vi "Generate Unique Random Name.vi"(8 "error in (no error)":errorcluster, 11 "Main in":refnum<class "Main.lvclass">) -> (0 "error out":errorcluster, 2 "Name":string, 3 "Main out":refnum<class "Main.lvclass">)   [LabVIEW 2020, in "Main.lvclass"]
uses:
  Main.lvclass
  Main.lvclass/Main.ctl
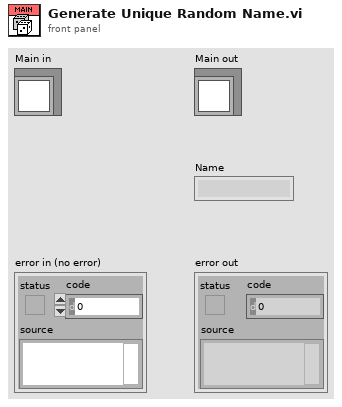
[diagram p1: front panel]
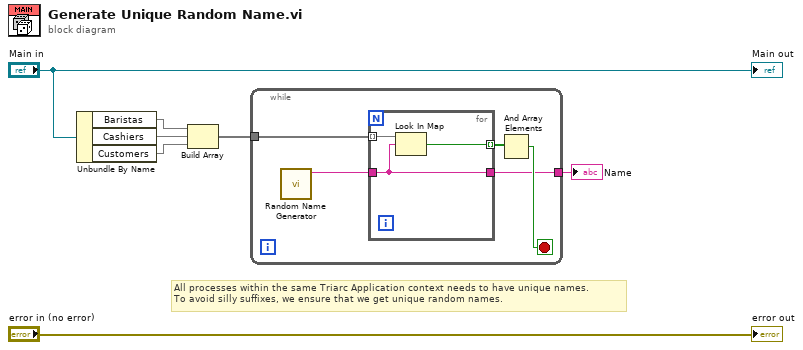
[diagram p0: block diagram]
diagram:
  # "All processes within the same Triarc Application context needs to have unique names.\nTo avoid silly suffixes, we ensure that we get unique random names."
  n1 = Unbundle By Name("Main in") -> ("Baristas"=w5:map{string, string}, "Cashiers"=w4:map{string, string}, "Customers"=w3:map{string, string})
  n2 = Build Array(w5, w4, w3) -> (w2:map{string, string}[])
  n3 = while {
    tunnel: w2 -> [w12]
    tunnel: [w8] -> w1
    stop <- w9 stop-if-true
    n4 = call "Random Name Generator.vi"() -> ("Name"=w11:string)  [unwired: 11 in]
    n5 = for {
      tunnel: w12 -> [w15] mode=indexing
      tunnel: w11 -> [w13]
      tunnel: [w14] -> w10 mode=indexing
      tunnel: [w13] -> w8
      n6 = Look In Map(map=w15, key=w13) -> (key not found?=w14:bool)  [unwired: 1 in, 1 out]
    }
    n7 = And Array Elements(Boolean array=w10) -> (logical AND=w9:bool)
  }
  "Name" <- w1
  "error out" <- "error in (no error)"
  "Main out" <- "Main in"
